vi "senser.vi"(1 "待处理数据":u8[](array[numeric])) -> (0 "输出簇":T1)   [LabVIEW 2014]
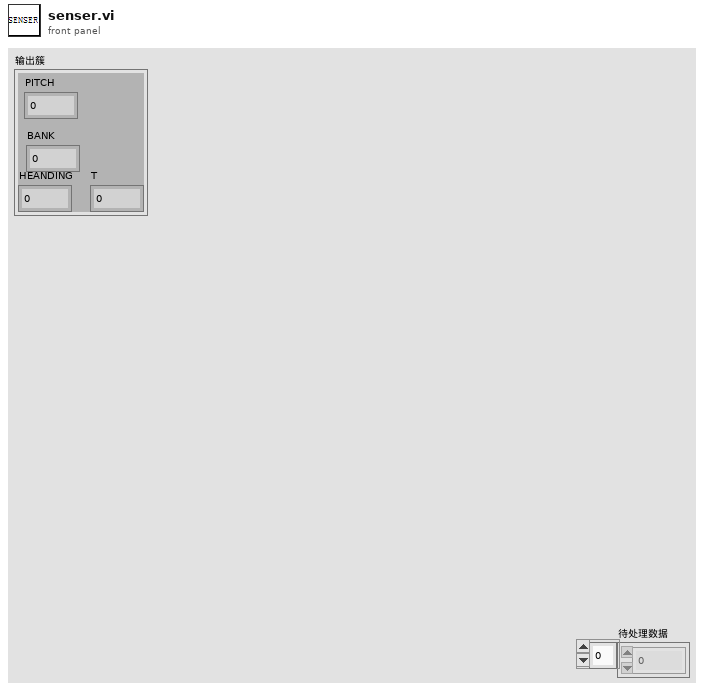
[diagram p1: front panel]
types:
  T1 = cluster{"PITCH":i32, "BANK":i32, "HEANDING":i32, "T":i32}
  T2 = cluster{"16位整型":u16, "16位整型":u16, "16位整型":u16, "16位整型":u16}
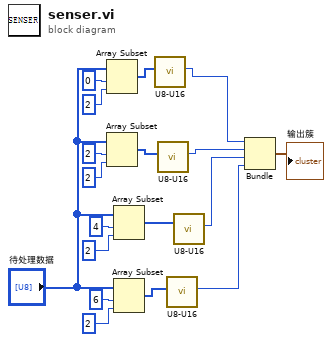
[diagram p0: block diagram]
diagram:
  n1 = Array Subset(array="待处理数据", index=0 ("长度（剩余）"), length=2 ("长度（剩余）")) -> (w8:u8[])
  n2 = Array Subset(array="待处理数据", index=2 ("长度（剩余）"), length=2 ("长度（剩余）")) -> (w5:u8[])
  n3 = Array Subset(array="待处理数据", index=4 ("长度（剩余）"), length=2 ("长度（剩余）")) -> (w4:u8[])
  n4 = Array Subset(array="待处理数据", index=6 ("长度（剩余）"), length=2 ("长度（剩余）")) -> (w2:u8[])
  n5 = call "U8-U16.vi"("数组"=w8) -> ("16位整型"=w7:u16)  [unwired: 8 in, 1 out]
  n6 = call "U8-U16.vi"("数组"=w5) -> ("16位整型"=w6:u16)  [unwired: 8 in, 1 out]
  n7 = call "U8-U16.vi"("数组"=w2) -> ("16位整型"=w1:u16)  [unwired: 8 in, 1 out]
  n8 = call "U8-U16.vi"("数组"=w4) -> ("16位整型"=w3:u16)  [unwired: 8 in, 1 out]
  n9 = Bundle("16位整型"=w7, "16位整型"=w6, "16位整型"=w3, "16位整型"=w1) -> (→"输出簇":T2)  [unwired: 1 in]
